vi "Add Core Dependencies.vi"(8 "error in (no error)":errorcluster, 11 "Item Ref in":T1 format="%.0x") -> (0 "error out":errorcluster, 3 "Device Ref out":T1 format="%.0x")   [LabVIEW 2020, in "DSF System Explorer.lvlib"]
uses:
  DSF System Explorer.lvlib
  <vilib>/NI VeriStand/Custom Device API/Custom Device Item Ref.ctl
  <vilib>/NI VeriStand/Custom Device API/Custom Device File Dependency.ctl
  <vilib>/NI VeriStand/Custom Device API/Path Specification.ctl
  <vilib>/NI VeriStand/Custom Device API/Path Type.ctl
  <vilib>/NI VeriStand/Custom Device API/Custom Device Supported Target.ctl
  <vilib>/NI VeriStand/Custom Device API/Custom Device API.lvlib
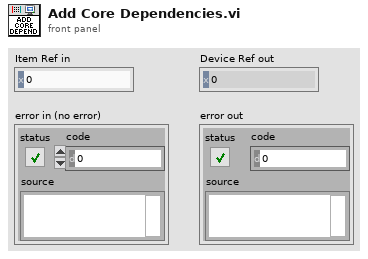
[diagram p1: front panel]
types:
  T1 = typedef "Custom Device API.lvlib/Custom Device Item Ref.ctl" = u64
  T2 = typedef "Custom Device API.lvlib/Custom Device Target Type.ctl" = enum16{"PharLap", "VxWorks", "Windows", "Linux_32_ARM", "Linux_x64"}
  T3 = typedef "Custom Device API.lvlib/Custom Device Supported Target.ctl" = enum16{"All", "PharLap", "VxWorks", "Windows", "Linux_32_ARM", "Linux_x64", "PharLap & Windows", "PharLap & VxWorks", "VxWorks & Windows"}
  T4 = typedef "Custom Device API.lvlib/Path Type.ctl" = enum16{"Absolute", "To Base", "To Common Data Dir", "To Application Data Dir"}
  T5 = typedef "Custom Device API.lvlib/Custom Device File Dependency.ctl" = cluster{"Source":T6, "RT Destination":path, "ForceDownload?":bool, "SupportedTarget":T3, "Version":string}
  T6 = typedef "Custom Device API.lvlib/Path Specification.ctl" = cluster{"Path":path, "Type":T4}
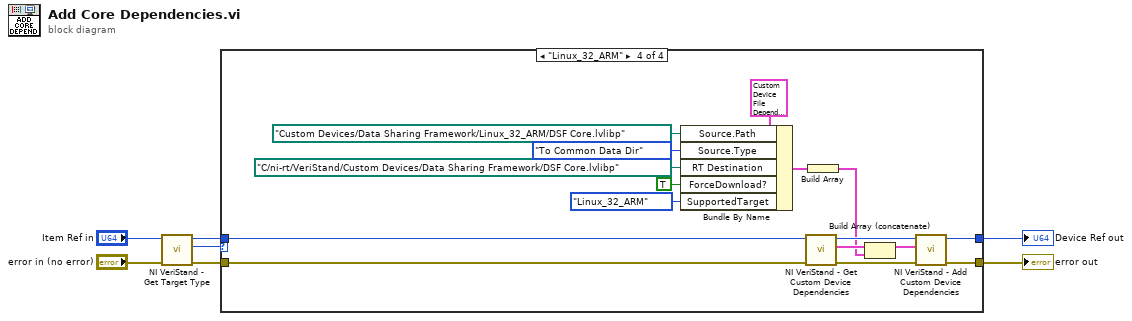
[diagram p0: block diagram]
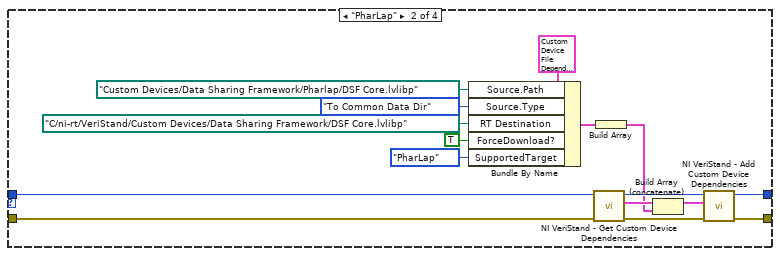
[diagram p3: hidden frame]
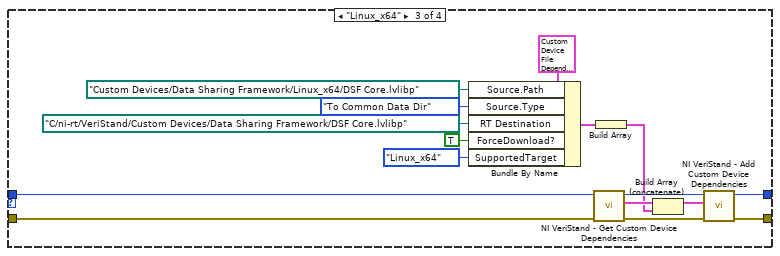
[diagram p4: hidden frame]
diagram:
  n1 = call <vilib>:"NI VeriStand - Get Target Type.vi"("error in (no error)"="error in (no error)", "Item Ref in"="Item Ref in") -> ("error out"=w6:errorcluster, "Target Type"=w7:T2, "Item Ref out"=w5:T1)  [unwired: 7 in]
  n2 = case shown="\"Linux_32_ARM\"" w7 {
    tunnel: [w9 w12 w28 w44] -> w1
    tunnel: [w8 w11 w27 w43] -> w2
    tunnel: w5 -> [w8 w13 w29 w45]
    tunnel: w6 -> [w9 w14 w30 w46]
    frame "Windows", Default {
      # "Don't add dependency for Windows or unsupported target type."
    }
    frame "PharLap" {
      n3 = Bundle By Name(cluster=T5 {"Source"={"Path"=path "", "Type"=enum."Absolute"}, "RT Destination"=path "", "ForceDownload?"=FALSE, "SupportedTarget"=enum."PharLap", "Version"=""} ("Dependencies"), "Source.Path"=path "Custom Devices/Data Sharing Framework/Pharlap/DSF Core.lvlibp", "Source.Type"=Path_Type."To Common Data Dir", "RT Destination"=path "C:/ni-rt/VeriStand/Custom Devices/Data Sharing Framework/DSF Core.lvlibp", "ForceDownload?"=TRUE, "SupportedTarget"=Custom_Device_Supported_Target."PharLap") -> (w19:T5)
      n4 = call <vilib>:"NI VeriStand - Get Custom Device Dependencies.vi"("error in (no error)"=w14, "Device Ref in"=w13) -> ("error out"=w17:errorcluster, "Dependencies"=w18:T5[], "Device Ref out"=w15:T1)  [unwired: 7 in]
      n5 = Build Array(w19) -> (w10:T5[])
      n6 = Build Array (concatenate)(w18, w10) -> (w16:T5[])
      n7 = call <vilib>:"NI VeriStand - Add Custom Device Dependencies.vi"("error in (no error)"=w17, "Dependencies"=w16, "Device Ref in"=w15) -> ("error out"=w12:errorcluster, "Device Ref out"=w11:T1)  [unwired: 7 in]
    }
    frame "Linux_x64" {
      n8 = Bundle By Name(cluster=T5 {"Source"={"Path"=path "", "Type"=enum."Absolute"}, "RT Destination"=path "", "ForceDownload?"=FALSE, "SupportedTarget"=enum."PharLap", "Version"=""} ("Dependencies"), "Source.Path"=path "Custom Devices/Data Sharing Framework/Linux_x64/DSF Core.lvlibp", "Source.Type"=Path_Type."To Common Data Dir", "RT Destination"=path "C:/ni-rt/VeriStand/Custom Devices/Data Sharing Framework/DSF Core.lvlibp", "ForceDownload?"=TRUE, "SupportedTarget"=Custom_Device_Supported_Target."Linux_x64") -> (w35:T5)
      n9 = call <vilib>:"NI VeriStand - Get Custom Device Dependencies.vi"("error in (no error)"=w30, "Device Ref in"=w29) -> ("error out"=w33:errorcluster, "Dependencies"=w34:T5[], "Device Ref out"=w31:T1)  [unwired: 7 in]
      n10 = Build Array(w35) -> (w26:T5[])
      n11 = Build Array (concatenate)(w34, w26) -> (w32:T5[])
      n12 = call <vilib>:"NI VeriStand - Add Custom Device Dependencies.vi"("error in (no error)"=w33, "Dependencies"=w32, "Device Ref in"=w31) -> ("error out"=w28:errorcluster, "Device Ref out"=w27:T1)  [unwired: 7 in]
    }
    frame "Linux_32_ARM" {
      n13 = Bundle By Name(cluster=T5 {"Source"={"Path"=path "", "Type"=enum."Absolute"}, "RT Destination"=path "", "ForceDownload?"=FALSE, "SupportedTarget"=enum."PharLap", "Version"=""} ("Dependencies"), "Source.Path"=path "Custom Devices/Data Sharing Framework/Linux_32_ARM/DSF Core.lvlibp", "Source.Type"=Path_Type."To Common Data Dir", "RT Destination"=path "C:/ni-rt/VeriStand/Custom Devices/Data Sharing Framework/DSF Core.lvlibp", "ForceDownload?"=TRUE, "SupportedTarget"=Custom_Device_Supported_Target."Linux_32_ARM") -> (w51:T5)
      n14 = call <vilib>:"NI VeriStand - Get Custom Device Dependencies.vi"("error in (no error)"=w46, "Device Ref in"=w45) -> ("error out"=w49:errorcluster, "Dependencies"=w50:T5[], "Device Ref out"=w47:T1)  [unwired: 7 in]
      n15 = Build Array(w51) -> (w42:T5[])
      n16 = Build Array (concatenate)(w50, w42) -> (w48:T5[])
      n17 = call <vilib>:"NI VeriStand - Add Custom Device Dependencies.vi"("error in (no error)"=w49, "Dependencies"=w48, "Device Ref in"=w47) -> ("error out"=w44:errorcluster, "Device Ref out"=w43:T1)  [unwired: 7 in]
    }
  }
  "Device Ref out" <- w2
  "error out" <- w1
